vi "init Tests.vi"(8 "error in (no error)":errorcluster caption="Error in", 11 "Tektronix RSA5106A Eingang":refnum<class "Tektronix RSA5106A.lvclass"> caption="DNL_LabVIEW Object in") -> (0 "error out":errorcluster caption="Error out", 3 "Tektronix RSA5106A Ausgang":refnum<class "Tektronix RSA5106A.lvclass"> caption="DNL_LabVIEW Object out")   [LabVIEW 2013, in "Tektronix RSA5106A.lvclass"]
uses:
  Tektronix RSA5106A.lvclass
  Tests/Stoeraussendung/Stoeraussendung.lvclass
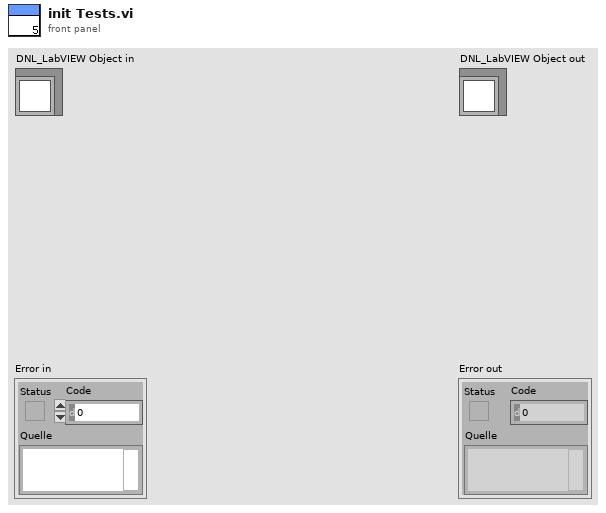
[diagram p1: front panel]
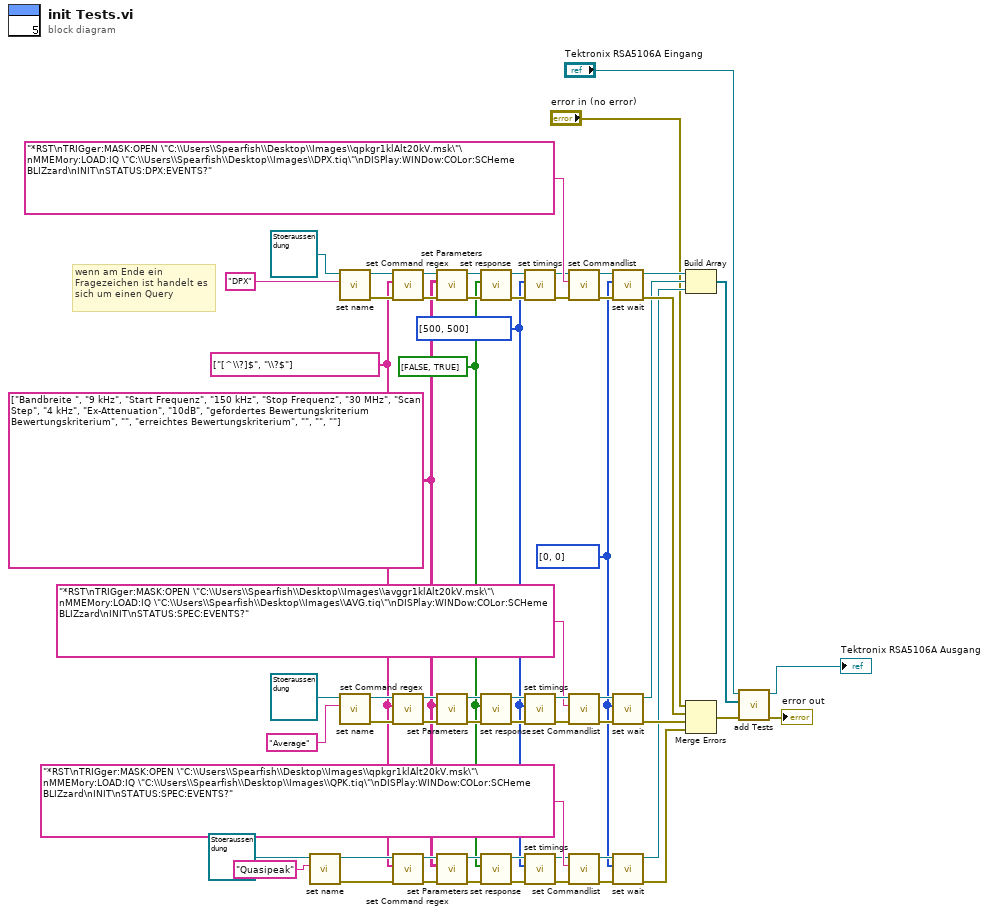
[diagram p0: block diagram]
diagram:
  w4 = u32[] [0, 0] ("wait")
  w1 = string[] ["[^\\?]$", "\\?$"] ("Command regex")
  w2 = bool[] [FALSE, TRUE] ("response?")
  w5 = string[][] [["Bandbreite ", "9 kHz"], ["Start Frequenz", "150 kHz"], ["Stop Frequenz", "30 MHz"], ["Scan Step", "4 kHz"], ["Ex-Attenuation", "10dB"], ["gefordertes Bewertungskriterium Bewertungskriterium", ""], ["erreichtes Bewertungskriterium", ""], ["", ""]] ("parameters")
  w3 = i32[] [500, 500] ("timings")
  # "wenn am Ende ein Fragezeichen ist handelt es sich um einen Query"
  n1 = call-dynamic "set name.vi"("name"="Quasipeak", "TestInterface (Eingang)"=refnum<class "Stoeraussendung.lvclass"> refnum ("Stoeraussendung.lvclass")) -> ("error out"=w25:errorcluster, "TestInterface (Ausgang)"=w23:refnum<class "Stoeraussendung.lvclass">)  [unwired: 8 in]
  n2 = call-dynamic "set name.vi"("name"="DPX", "TestInterface (Eingang)"=refnum<class "Stoeraussendung.lvclass"> refnum ("Stoeraussendung.lvclass")) -> ("error out"=w55:errorcluster, "TestInterface (Ausgang)"=w53:refnum<class "Stoeraussendung.lvclass">)  [unwired: 8 in]
  n3 = call-dynamic "set name.vi"("name"="Average", "TestInterface (Eingang)"=refnum<class "Stoeraussendung.lvclass"> refnum ("Stoeraussendung.lvclass")) -> ("error out"=w40:errorcluster, "TestInterface (Ausgang)"=w42:refnum<class "Stoeraussendung.lvclass">)  [unwired: 8 in]
  n4 = call-dynamic "set Command regex.vi"("error in (no error)"=w55, "Command regex"=w1, "TestInterface (Eingang)"=w53) -> ("error out"=w56:errorcluster, "TestInterface (Ausgang)"=w52:refnum<class "Stoeraussendung.lvclass">)  [unwired: 7 in]
  n5 = call-dynamic "set Command regex.vi"("error in (no error)"=w40, "Command regex"=w1, "TestInterface (Eingang)"=w42) -> ("error out"=w39:errorcluster, "TestInterface (Ausgang)"=w43:refnum<class "Stoeraussendung.lvclass">)  [unwired: 7 in]
  n6 = call-dynamic "set Command regex.vi"("error in (no error)"=w25, "Command regex"=w1, "TestInterface (Eingang)"=w23) -> ("error out"=w26:errorcluster, "TestInterface (Ausgang)"=w22:refnum<class "Stoeraussendung.lvclass">)  [unwired: 7 in]
  n7 = call-dynamic "set Parameters.vi"("error in (no error)"=w56, "parameters"=w5, "TestInterface (Eingang)"=w52) -> ("error out"=w57:errorcluster, "TestInterface (Ausgang)"=w51:refnum<class "Stoeraussendung.lvclass">)  [unwired: 7 in]
  n8 = call-dynamic "set Parameters.vi"("error in (no error)"=w39, "parameters"=w5, "TestInterface (Eingang)"=w43) -> ("error out"=w38:errorcluster, "TestInterface (Ausgang)"=w44:refnum<class "Stoeraussendung.lvclass">)  [unwired: 7 in]
  n9 = call-dynamic "set Parameters.vi"("error in (no error)"=w26, "parameters"=w5, "TestInterface (Eingang)"=w22) -> ("error out"=w27:errorcluster, "TestInterface (Ausgang)"=w21:refnum<class "Stoeraussendung.lvclass">)  [unwired: 7 in]
  n10 = call-dynamic "set response.vi"("error in (no error)"=w57, "response?"=w2, "TestInterface (Eingang)"=w51) -> ("error out"=w58:errorcluster, "TestInterface (Ausgang)"=w50:refnum<class "Stoeraussendung.lvclass">)  [unwired: 7 in]
  n11 = call-dynamic "set response.vi"("error in (no error)"=w38, "response?"=w2, "TestInterface (Eingang)"=w44) -> ("error out"=w37:errorcluster, "TestInterface (Ausgang)"=w45:refnum<class "Stoeraussendung.lvclass">)  [unwired: 7 in]
  n12 = call-dynamic "set response.vi"("error in (no error)"=w27, "response?"=w2, "TestInterface (Eingang)"=w21) -> ("error out"=w28:errorcluster, "TestInterface (Ausgang)"=w20:refnum<class "Stoeraussendung.lvclass">)  [unwired: 7 in]
  n13 = call-dynamic "set timings.vi"("error in (no error)"=w58, "timings"=w3, "TestInterface (Eingang)"=w50) -> ("error out"=w59:errorcluster, "TestInterface (Ausgang)"=w54:refnum<class "Stoeraussendung.lvclass">)  [unwired: 7 in]
  n14 = call-dynamic "set timings.vi"("error in (no error)"=w37, "timings"=w3, "TestInterface (Eingang)"=w45) -> ("error out"=w36:errorcluster, "TestInterface (Ausgang)"=w41:refnum<class "Stoeraussendung.lvclass">)  [unwired: 7 in]
  n15 = call-dynamic "set timings.vi"("error in (no error)"=w28, "timings"=w3, "TestInterface (Eingang)"=w20) -> ("error out"=w29:errorcluster, "TestInterface (Ausgang)"=w24:refnum<class "Stoeraussendung.lvclass">)  [unwired: 7 in]
  n16 = call-dynamic "set Commandlist.vi"("error in (no error)"=w59, "Commandlist"="*RST\nTRIGger:MASK:OPEN \"C:\\Users\\Spearfish\\Desktop\\Images\\qpkgr1klAlt20kV.msk\"\nMMEMory:LOAD:IQ \"C:\\Users\\Spearfish\\Desktop\\Images\\DPX.tiq\"\nDISPlay:WINDow:COLor:SCHeme BLIZzard\nINIT\nSTATUS:DPX:EVENTS?", "TestInterface (Eingang)"=w54) -> ("error out"=w60:errorcluster, "TestInterface (Ausgang)"=w61:refnum<class "Stoeraussendung.lvclass">)  [unwired: 7 in]
  n17 = call-dynamic "set Commandlist.vi"("error in (no error)"=w36, "Commandlist"="*RST\nTRIGger:MASK:OPEN \"C:\\Users\\Spearfish\\Desktop\\Images\\avggr1klAlt20kV.msk\"\nMMEMory:LOAD:IQ \"C:\\Users\\Spearfish\\Desktop\\Images\\AVG.tiq\"\nDISPlay:WINDow:COLor:SCHeme BLIZzard\nINIT\nSTATUS:SPEC:EVENTS?", "TestInterface (Eingang)"=w41) -> ("error out"=w35:errorcluster, "TestInterface (Ausgang)"=w34:refnum<class "Stoeraussendung.lvclass">)  [unwired: 7 in]
  n18 = call-dynamic "set Commandlist.vi"("error in (no error)"=w29, "Commandlist"="*RST\nTRIGger:MASK:OPEN \"C:\\Users\\Spearfish\\Desktop\\Images\\qpkgr1klAlt20kV.msk\"\nMMEMory:LOAD:IQ \"C:\\Users\\Spearfish\\Desktop\\Images\\QPK.tiq\"\nDISPlay:WINDow:COLor:SCHeme BLIZzard\nINIT\nSTATUS:SPEC:EVENTS?", "TestInterface (Eingang)"=w24) -> ("error out"=w30:errorcluster, "TestInterface (Ausgang)"=w31:refnum<class "Stoeraussendung.lvclass">)  [unwired: 7 in]
  n19 = call-dynamic "set wait.vi"("error in (no error)"=w60, "wait"=w4, "TestInterface in"=w61) -> ("error out"=w17:errorcluster, "TestInterface out"=w14:refnum<class "Stoeraussendung.lvclass">)  [unwired: 7 in]
  n20 = call-dynamic "set wait.vi"("error in (no error)"=w35, "wait"=w4, "TestInterface in"=w34) -> ("error out"=w16:errorcluster, "TestInterface out"=w13:refnum<class "Stoeraussendung.lvclass">)  [unwired: 7 in]
  n21 = call-dynamic "set wait.vi"("error in (no error)"=w30, "wait"=w4, "TestInterface in"=w31) -> ("error out"=w15:errorcluster, "TestInterface out"=w12:refnum<class "Stoeraussendung.lvclass">)  [unwired: 7 in]
  n22 = Build Array(w14, w13, w12) -> (w11:refnum<class "Stoeraussendung.lvclass">[])
  n23 = Merge Errors("error in (no error)", w17, w16, w15) -> (w8:errorcluster)
  n24 = call-dynamic "add Tests.vi"("error in (no error)"=w8, "Tests"=w11, "DeviceInterface (Eingang)"="Tektronix RSA5106A Eingang") -> ("error out"=→"error out":errorcluster, "DeviceInterface (Ausgang)"=→"Tektronix RSA5106A Ausgang":refnum<class "Tektronix RSA5106A.lvclass">)  [unwired: 7 in]
